vi "Modulus.vi"(1 "Input":cluster{"Input value":dbl, "Base":dbl} {"Base" format="%.2f"; "Input value" format="%.2f"}) -> (0 "Output":T1 {"Number of\nComplete Cycles" format="%.2f"; "Modulus" format="%.2f"})   [LabVIEW 2022 SP3]
panel:
  # "This VI Computes the Modulus Function"
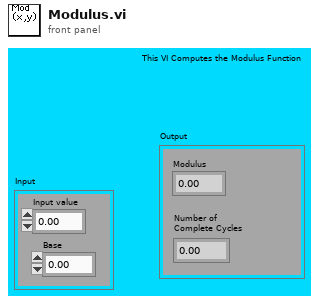
[diagram p1: front panel]
types:
  T1 = cluster{"Modulus":dbl, "Number of\nComplete Cycles":dbl}
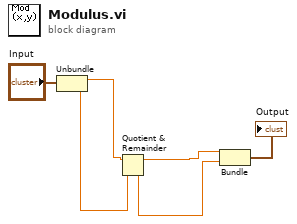
[diagram p0: block diagram]
diagram:
  n1 = Unbundle("Input") -> ("Input value"=w5:dbl, "Base"=w4:dbl)
  n2 = Quotient & Remainder(x=w5, y=w4) -> (x-y*floor(x/y)=w3:dbl, floor(x/y)=w1:dbl)
  n3 = Bundle(w3, w1) -> (→"Output":cluster{dbl, dbl})  [unwired: 1 in]
